vi "keyboardTester.vi"() -> ()   [LabVIEW 2018]
uses:
  <vilib>/Utility/inputDevices.llb/keyboardAcquire.vi
  <vilib>/Utility/inputDevices.llb/closeKeyboard.vi
panel:
  out "rc command":string
  out "yaw, up/down":cluster{dbl[], dbl[]}(graph)
  out "left/right, back/forward":cluster{dbl[], dbl[]}(graph)
  in  "stop":bool
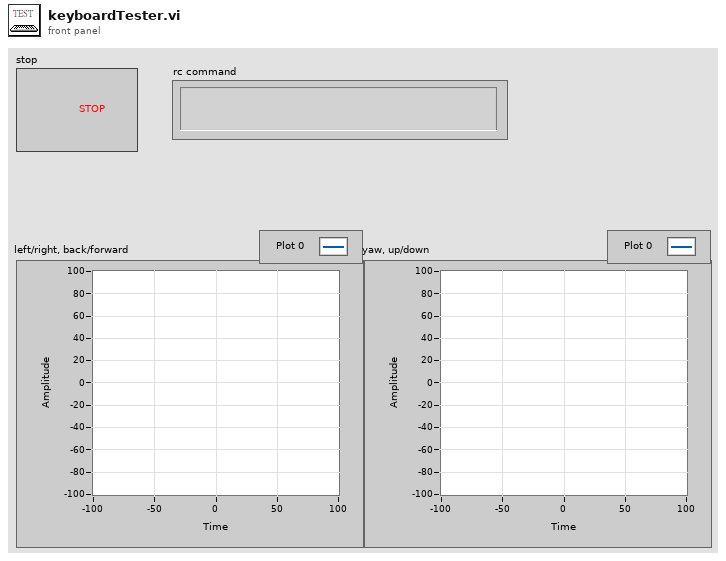
[diagram p1: front panel]
types:
  T1 = enum16{"0", "1", "2", "3", "4", "5", "6", "7", "8", "9", "A", "B", "C", "D", "E", "F", "G", "H", "I", "J", "K", "L", "M", "N", "O", "P", "Q", "R", "S", "T", "U", "V", "W", "X", "Y", "Z", "F1", "F2", "F3", "F4", "F5", "F6", "F7", "F8", "F9", "F10", "F11", "F12", "F13", "F14", "F15", "ADD", "BACK", "BACKSLASH", "CAPITAL", "COMMA", "DECIMAL", "DELETE", "DIVIDE", "DOWN", "END", "EQUALS", "ESCAPE", "GRAVE (`)", "HOME", "INSERT", "LBRACKET", "LCONTROL", "LEFT", "L ALT", "LSHIFT", "LWIN", "MINUS", "MULTIPLY", "NEXT", "NUMLOCK", "NUMPAD_0", "NUMPAD_1", "NUMPAD_2", "NUMPAD_3", "NUMPAD_4", "NUMPAD_5", "NUMPAD_6", "NUMPAD_7", "NUMPAD_8", "NUMPAD_9", "PAUSE", "PERIOD", "PRIOR (PG UP)", "RBRACKET", "RCONTROL", "RETURN", "RIGHT", "R ALT", "RSHIFT", "RWIN", "SCROLL", "SEMICOLON", "SLASH", "SPACE", "SUBTRACT", "TAB", "UP", "ENTER (num pad)", "' (quote)"}
  T2 = enum16{"0", "1", "2", "3", "4", "5", "6", "7", "8", "9", "A", "B", "C", "D", "E", "F", "G", "H", "I", "J", "K", "L", "M", "N", "O", "P", "Q", "R", "S", "T", "U", "V", "W", "X", "Y", "Z", "F1", "F2", "F3", "F4", "F5", "F6", "F7", "F8", "F9", "F10", "F11", "F12", "F13", "F14", "F15", "ADD", "BACK", "BACKSLASH", "CAPITAL", "COMMA", "DECIMAL", "DELETE", "DIVIDE", "DOWN", "END", "EQUALS", "ESCAPE", "GRAVE (`)", "HOME", "INSERT", "LBRACKET", "LCONTROL", "LEFT", "L ALT", "LSHIFT", "LWIN", "MINUS", "MULTIPLY", "NEXT", "NUMLOCK", "NUMPAD_0", "NUMPAD_1", "NUMPAD_2", "NUMPAD_3", "NUMPAD_4", "NUMPAD_5", "NUMPAD_6", "NUMPAD_7", "NUMPAD_8", "NUMPAD_9", "PAUSE", "PERIOD", "PRIOR (PG UP)", "RBRACKET", "RCONTROL", "RETURN", "RIGHT", "R ALT", "RSHIFT", "RWIN", "SCROLL", "SEMICOLON", "SLASH", "SPACE", "SUBTRACT", "TAB", "UP", "ENTER (num pad)", "' (quote)"}[]
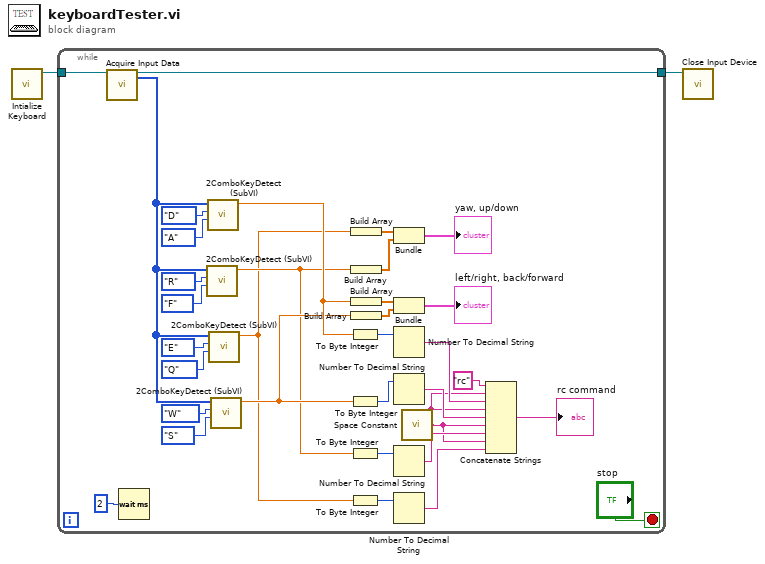
[diagram p0: block diagram]
diagram:
  n1 = call <vilib>:"Intialize Keyboard.vi"() -> ("device ID"=w2:refnum<k1>)  [unwired: 10 in, 1 out]
  n2 = while {
    tunnel: w2 -> [w36]
    tunnel: [w26] -> w1
    stop <- "stop" stop-if-true
    n3 = call-poly <vilib>:"Acquire Input Data.vi"("device ID"=w36) -> ("device ID"=w26:refnum<k1>, "keys pressed"=w21:T2)  [unwired: 16 in, 1 out]
    n4 = Wait (ms)(milliseconds to wait=u32 2) -> ()  [unwired: 1 out]
    n5 = call "2ComboKeyDetect (SubVI).vi"("negKey"=T1."F" ("element"), "posKey"=T1."R" ("element"), "keys pressed"=w21) -> ("speedout"=w15:dbl)  [unwired: 8 in]
    n6 = call "2ComboKeyDetect (SubVI).vi"("negKey"=T1."A" ("element"), "posKey"=T1."D" ("element"), "keys pressed"=w21) -> ("speedout"=w17:dbl)  [unwired: 8 in]
    n7 = call "2ComboKeyDetect (SubVI).vi"("negKey"=T1."Q" ("element"), "posKey"=T1."E" ("element"), "keys pressed"=w21) -> ("speedout"=w14:dbl)  [unwired: 8 in]
    n8 = call "2ComboKeyDetect (SubVI).vi"("negKey"=T1."S" ("element"), "posKey"=T1."W" ("element"), "keys pressed"=w21) -> ("speedout"=w16:dbl)  [unwired: 8 in]
    n9 = To Byte Integer(number=w17) -> (8bit integer=w12:i8)
    n10 = To Byte Integer(number=w16) -> (8bit integer=w10:i8)
    n11 = To Byte Integer(number=w15) -> (8bit integer=w8:i8)
    n12 = To Byte Integer(number=w14) -> (8bit integer=w4:i8)
    n13 = Build Array(w14) -> (w20:dbl[])
    n14 = Build Array(w15) -> (w19:dbl[])
    n15 = Build Array(w17) -> (w30:dbl[])
    n16 = Build Array(w16) -> (w29:dbl[])
    n17 = Bundle(w20, w19) -> (→"yaw, up/down":cluster{dbl[], dbl[]})  [unwired: 1 in]
    n18 = Bundle(w30, w29) -> (→"left/right, back/forward":cluster{dbl[], dbl[]})  [unwired: 1 in]
    n19 = Number To Decimal String(number=w12) -> (decimal integer string=w11:string)  [unwired: 1 in]
    n20 = Number To Decimal String(number=w10) -> (decimal integer string=w9:string)  [unwired: 1 in]
    n21 = Number To Decimal String(number=w8) -> (decimal integer string=w7:string)  [unwired: 1 in]
    n22 = Number To Decimal String(number=w4) -> (decimal integer string=w5:string)  [unwired: 1 in]
    n23 = call <vilib>:"Space Constant.vi"() -> ("String"=w6:string)
    n24 = Concatenate Strings("rc" ("string"), w6, w11, w6, w9, w6, w7, w6, w5) -> (→"rc command":string)
  }
  n25 = call-poly <vilib>:"Close Input Device.vi"("device ID"=w1) -> ()  [unwired: 9 in, 1 out]
